vi "user32_LoadImage.vi"(0 "hInst":u32, 1 "uType":u32(ring) items=["BITMAP", "ICON", "CURSOR"], 5 "ImagePath":path, 7 "Size":cluster{"Width":i32, "Height":i32}, 9 "fuLoad":u32(ring) items=["DEFAULTCOLOR"=0, "MONOCHROME"=1, "LOADFROMFILE"=16, "LOADTRANSPARENT"=32, "DEFAULTSIZE"=64, "DEFAULTSIZE"=128, "LOADMAP3DCOLORS"=4096, "CREATEDIBSECTION"=8192, "SHARED"=32768], 11 "错误输入（无错误）":errorcluster) -> (4 "dup hInst":u32, 15 "错误输出":errorcluster)   [LabVIEW 2011]
doc: "该函数装载图标，光标，或位图。"
uses:
  user32.dll
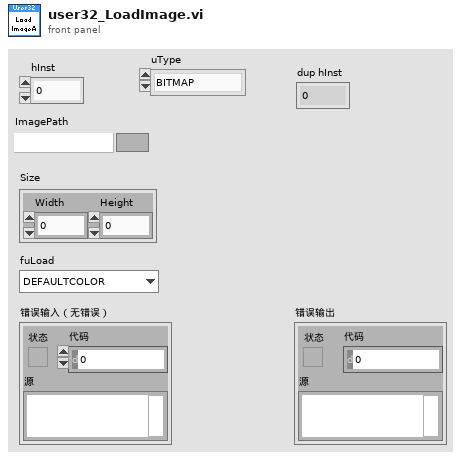
[diagram p1: front panel]
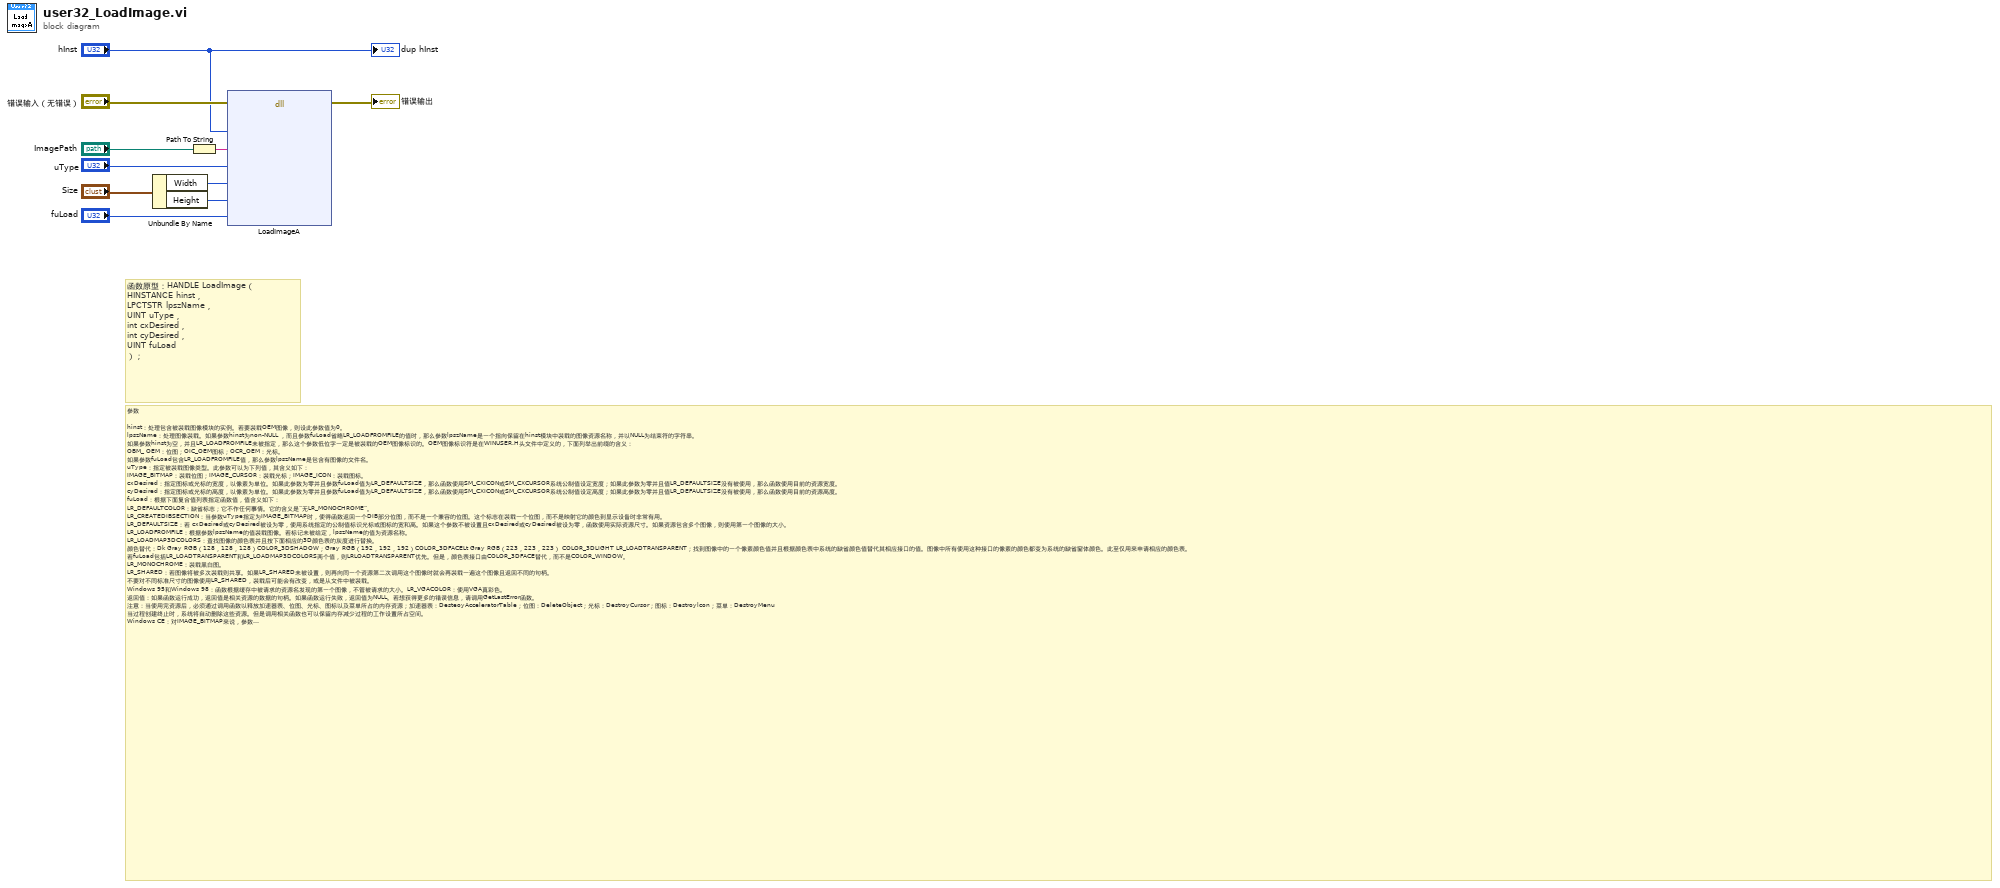
[diagram p0: block diagram]
diagram:
  # "参数\n\nhinst：处理包含被装载图像模块的实例。若要装载OEM图像，则设此参数值为0。\nlpszName：处理图像装载。如果参数hinst为non-NULL ，而且参数fuLoad省略LR_LOADFROMFILE的值时，那么参数lpszName是一个指向保留在hinst模块中装载的图像资源名称，并以NULL为结束符的字符串。\n如果参数hinst为空，并且LR_LOADFROMFILE未被指定，那么这个参数低位字一定是被装载的OEM图像标识的。OEM图像标识符是在WINUSER.H头文件中定义的，下面列举出前缀的含义：\nOBM_ OEM：位图；OIC_OEM图标；OCR_OEM：光标。\n如果参数fuLoad包含LR_LOADFROMFILE值，那么参数lpszName是包含有图像的文件名。\nuType：指定被装载图像类型。此参数可以为下列值，其含义如下：\nIMAGE_BITMAP：装载位图；IMAGE_CURSOR：装载光标；IMAGE_ICON：装载图标。\ncxDesired：指定图标或光标的宽度，以像素为单位。如果此参数为零并且参数fuLoad值为LR_DEFAULTSIZE，那么函数使用SM_CXICON或SM_CXCURSOR系统公制值设定宽度；如果此参数为零并且值LR_DEFAULTSIZE没有被使用，那么函数使用目前的资源宽度。\ncyDesired：指定图标或光标的高度，以像素为单位。如果此参数为零并且参数fuLoad值为LR_DEFAULTSIZE，那么函数使用SM_CXICON或SM_CXCURSOR系统公制值设定高度；如果此参数为零并且值LR_DEFAULTSIZE没有被使用，那么函数使用目前的资源高度。\nfuLoad：根据下面复合值列表指定函数值，值含义如下：\nLR_DEFAULTCOLOR：缺省标志；它不作任何事情。它的含义是“无LR_MONOCHROME”。\nLR_CREATEDIBSECTION：当参数uType指定为IMAGE_BITMAP时，使得函数返回一个DIB部分位图，而不是一个兼容的位图。这个标志在装载一个位图，而不是映射它的颜色到显示设备时非常有用。\nLR_DEFAULTSIZE：若 cxDesired或cyDesired被设为零，使用系统指定的公制值标识光标或图标的宽和高。如果这个参数不被设置且cxDesired或cyDesired被设为零，函数使用实际资源尺寸。如果资源包含多个图像，则使用第一个图像的大小。\nLR_LOADFROMFILE：根据参数lpszName的值装载图像。若标记未被给定，lpszName的值为资源名称。\nLR_LOADMAP3DCOLORS：查找图像的颜色表并且按下面相应的3D颜色表的灰度进行替换。\n颜色替代：Dk Gray RGB（128，128，128）COLOR_3DSHADOW；Gray RGB（192，192，192）COLOR_3DFACELt Gray RGB（223，223，223） COLOR_3DLIGHT LR_LOADTRANSPARENT；找到图像中的一个像素颜色值并且根据颜色表中系统的缺省颜色值替代其相应接口的值。图像中所有使用这种接口的像素的颜色都变为系统的缺省窗体颜色。此至仅用来申请相应的颜色表。\n若fuLoad包括LR_LOADTRANSPARENT和LR_LOADMAP3DCOLORS两个值，则LRLOADTRANSPARENT优先。但是，颜色表接口由COLOR_3DFACE替代，而不是COLOR_WINDOW。\nLR_MONOCHROME：装载黑白图。\nLR_SHARED：若图像将被多次装载则共享。如果LR_SHARED未被设置，则再向同一个资源第二次调用这个图像时就会再装载一遍这个图像且返回不同的句柄。\n不要对不同标准尺寸的图像使用LR_SHARED，装载后可能会有改变，或是从文件中被装载。\nWindows 95和Windows 98：函数根据缓存中被请求的资源名发现的第一个图像，不管被请求的大小。LR_VGACOLOR：使用VGA真彩色。\n返回值：如果函数运行成功，返回值是相关资源的数据的句柄。如果函数运行失败，返回值为NULL。若想获得更多的错误信息，请调用GetLastError函数。\n注意：当使用完资源后，必须通过调用函数以释放加速器表、位图、光标、图标以及菜单所占的内存资源；加速器表：DesteoyAcceleratorTable；位图：DeleteObject；光标：DestroyCursor；图标：Destroylcon；菜单：DestroyMenu\n当过程创建终止时，系统将自动删除这些资源。但是调用相关函数也可以保留内存减少过程的工作设置所占空间。\nWindows CE：对IMAGE_BITMAP来说，参数cxDesred和cyDesred p必须为零。Windows CE不支持图表跳跃或闪烁。\n参数fuLoad必须为（=LR_DEFAULTCOLOR）。\n如果的目标平台不支持鼠标光标，可以指定在参数cxDesred和cyDsired的SM_CXCURSOR和SM_CYCURSOR的值，但不能指定参数uType中IMAGE_CURSOR的值。\n如果目标平台支持鼠标光标，可以指定在参数cxDesired和cyDesred的SM_CXCURSOR和SM_CYCURSOR的值，也能指定参数uType中IMAGE_CURSOR的值。\n函数说明：该函数不可用来装载jpg等格式图片，可使用gdi+函数GdipDrawImage装在jpg，png等格式图片"
  # "函数原型：HANDLE LoadImage（\nHINSTANCE hinst，\nLPCTSTR lpszName，\nUINT uType，\nint cxDesired，\nint cyDesired，\nUINT fuLoad\n）；"
  n1 = Unbundle By Name("Size") -> ("Width"=w5:i32, "Height"=w4:i32)
  n2 = Path To String(path="ImagePath") -> (string=w1:string)
  n3 = dll-call lib="user32.dll" fn="LoadImageA"(error in="错误输入（无错误）", "hInst"="hInst", "lpszName"=w1, "uType"="uType", "cxDesired"=w5, "cyDesired"=w4, "fuLoad"="fuLoad") -> (error out=→"错误输出":errorcluster)  [unwired: 9 in, 1 out]
  "dup hInst" <- "hInst"
